vi "SUB_Write File+ (string).vi"(4 "convert eol? (no:F)":bool caption="eol 변환? (아니오:거짓)", 5 "string":string caption="문자열", 6 "error in (no error)":errorcluster caption="에러 입력(에러 없음)", 7 "pos offset (bytes:0)":i32 caption="위치 오프셋(바이트:0)", 8 "pos mode (rel. to end:1)":enum16{"start", "end", "current"}(ring)=enum."end" caption="위치 모드(끝 위치에 상대적:1)", 9 "refnum":refnum<file> caption="참조 번호") -> (0 "error out":errorcluster caption="에러 출력", 1 "mark after write (bytes)":i32 caption="쓰기 이후 마크(바이트)", 3 "dup refnum":refnum<file> caption="참조 번호 복제")   [LabVIEW 2015]
doc: "지정된 위치의 바이트 스트림 파일에 문자의 문자열을 씁니다; 기본 위치는 현재 마크입니다. VI는 전달되는 에러와 내부의 에러를 검사하고 에러가 발생되어 전달되면 쓰지 않습니다.\n\n참조 번호는 열린 파일의 참조 번호입니다.\n\n위치 모드는 위치 오프셋을 기준으로 쓰기의 시작 위치를 지정합니다:\n\n 0: 파일의 시작 위치 더하기 위치 오프셋.\n\n 1: 파일 끝 위치 더하기 위치 오프셋. 이것은 기본값입니다.\n\n 2: 현재 파일 마크 더하기 위치 오프셋.\n\n위치 오프셋은 동작 시작 후 위치 모드에 의해서 얼마나 먼 위치가 지정되었는지를 바이트로 지정합니다. 기본값은 0입니다.\n\n캐릭터 문자열은 VI가 파일에 쓰는 데이터입니다.\n\nLabVIEW 라인의 끝 마커를 플랫폼에 특정한 마커로 변환하기 위해서 eol 변환을 참으로 설정하십시오. 아무것도 하지 않기 위해서는 거짓(기본)으로 설정하십시오.\n\n에러 입력은 3개의 원소(에러?, 코드 그리고 소스)로 구성된 클러스터로 업스트림 에러 상태, 즉, VI의 실행을 처리중 발생한 모든 에러의 존재를 나타냅니다. VI는 오직 에러가 발생하지 않을 때에만 정상적으로 실행됩니다. 그렇지 않은 경우 VI는 에러 입력을 에러 출력으로 전달합니다. 에러?는 에러가 발생했을 경우 참입니다. 기본값은 거짓입니다. 코드는 에러 코드입니다; 기본값은 0입니다. 소스는 대부분의 경우 에러를 만든 VI 또는 함수의 이름입니다. 기본은 빈 문자열입니다.\n\n참조 번호 복제는 참조 번호와 같은 값을 가진 흐름 파라미터입니다.\n\n쓰기 이후의 마크는 마지막으로 쓴 문자 다음의 문자 위치입니다.\n\n에러 출력은 세가지 원소(에러?, 코드 그리고 소스)로 구성된 클러스터이며 VI 실행 중에 발생한 에러 상태를 나타냅니다. 만일 전달된 에러가 없다면, VI는 정상적으로 실행되고 에러 출력은 VI의 에러 상태를 나타냅니다; 만일 전달된 에러가 있다면, 에러 출력은 에러 입력과 동일합니다."
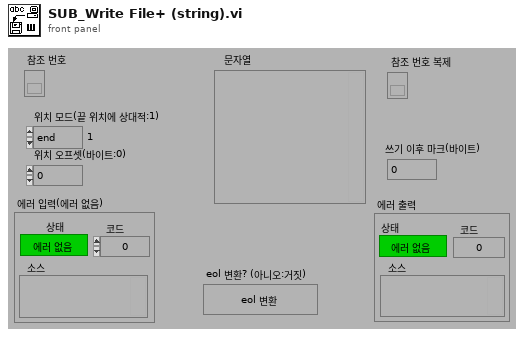
[diagram p1: front panel]
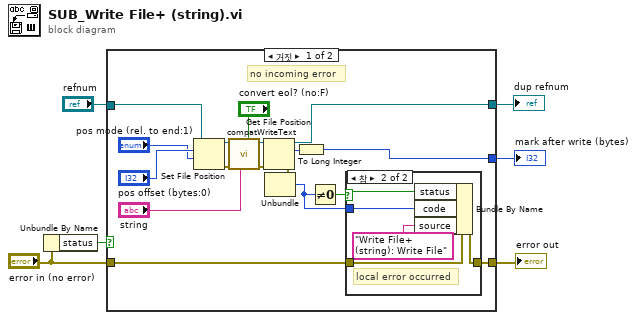
[diagram p0: block diagram]
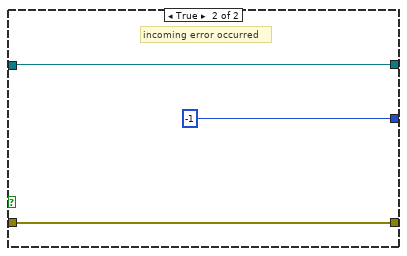
[diagram p3: hidden frame]
diagram:
  n1 = Unbundle By Name("error in (no error)") -> ("status"=w6:bool)
  n2 = case shown="거짓" w6 {
    tunnel: [w16 w31] -> w5
    tunnel: [w21 -1] -> w4
    tunnel: [w20 w30] -> w3
    tunnel: "refnum" -> [w19 w30]
    tunnel: "error in (no error)" -> [w15 w31]
    frame False {
      # "no incoming error"
      n3 = Set File Position(offset (in bytes) (0)="pos offset (bytes:0)", refnum=w19, from (0:start)="pos mode (rel. to end:1)") -> (refnum out=w11:refnum<file>, error out=w10:errorcluster)  [unwired: 1 in]
      n4 = call <vilib>:"compatWriteText.vi"("convert eol (F)"="convert eol? (no:F)", "data"="string", "error in"=w10, "refnum"=w11) -> ("error out"=w8:errorcluster, "dup refnum"=w9:refnum<file>)  [unwired: 6 in]
      n5 = Get File Position(4:w8, 7:w9) -> (0:w17:errorcluster, 2:w7:i64, 3:w20:refnum<file>)
      n6 = Unbundle(w17) -> ("code"=w13:i32)  [unwired: 2 out]
      n7 = To Long Integer(number=w7) -> (32bit integer=w21:i32)
      n8 = Not Equal To 0?(x=w13) -> (x != 0?=w14:bool)
      n9 = case shown="참" w14 {
        selector: w14 -> [_ w25]
        tunnel: w13 -> [_ w28]
        tunnel: [w24 w26] -> w16
        tunnel: w15 -> [w24 w27]
        frame False {
          # "no local error"
        }
        frame True {
          # "local error occurred"
          n10 = Bundle By Name(cluster=w27, "status"=w25, "code"=w28, "source"="Write File+ (string): Write File") -> (w26:errorcluster)
        }
      }
    }
    frame True {
      # "incoming error occurred"
    }
  }
  "error out" <- w5
  "mark after write (bytes)" <- w4
  "dup refnum" <- w3
